vi "testTestCaseExecuted.vi"() -> (0 "error out":errorcluster)   [LabVIEW 2017, in "TestSuite.Tests.lvlib" / "Run.lvlib"]
uses:
  Run.lvlib
  TestSuite/TestSuite.lvclass
  TestResult/TestResult.lvclass
  Support/TestCaseMock/TestCaseMock.lvclass
  C:/Users/de200256/Code/logmanoriginal/lvunit/Test/Test.lvclass
  Assertion/Assertion.lvlib
  Test/Test.lvclass
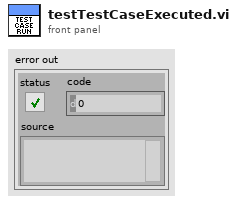
[diagram p1: front panel]
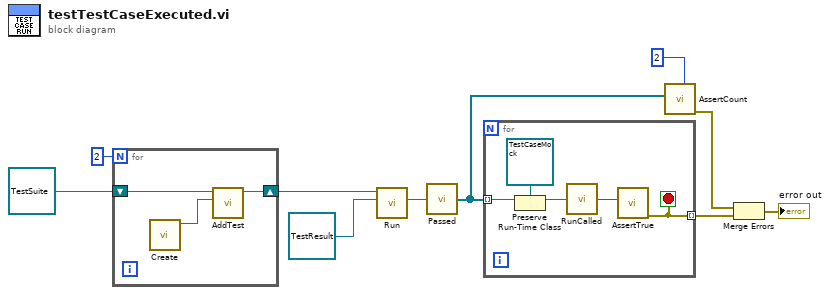
[diagram p0: block diagram]
diagram:
  n1 = for {
    N: 2 -> [_]
    shift-right: [w12] -> w8
    shift-left: refnum<class "TestSuite.lvclass"> refnum ("TestSuite.lvclass") -> [w13]
    n2 = call "Create.vi"() -> ("TestCaseMock"=w11:refnum<class "TestCaseMock.lvclass">)  [unwired: 10 in, 1 out]
    n3 = call-dynamic "AddTest.vi"("Test"=w11, "TestSuite in"=w13) -> ("TestSuite out"=w12:refnum<class "TestSuite.lvclass">)  [unwired: 8 in, 1 out]
  }
  n4 = call-dynamic "Run.vi"("TestResult"=refnum<class "TestResult.lvclass"> refnum ("TestResult.lvclass"), "TestSuite in"=w8) -> ("TestResult out"=w6:refnum<class "TestResult.lvclass">)  [unwired: 7 in, 2 out]
  n5 = call "Passed.vi"("TestResult In"=w6) -> ("Passed"=w2:refnum<class "Test.lvclass">[])
  n6 = for {
    tunnel: w2 -> [w18] mode=indexing
    tunnel: [w14] -> w5 mode=indexing
    stop <- w14 stop-if-true
    n7 = Preserve Run-Time Class(object in=w18, 2:refnum<class "TestCaseMock.lvclass"> refnum ("TestCaseMock")) -> (object out=w16:refnum<class "TestCaseMock.lvclass">)  [unwired: 1 in, 1 out]
    n8 = call "RunCalled.vi"("TestCaseMock In"=w16) -> ("Run Called"=w15:bool)
    n9 = call "AssertTrue.vi"("Condition"=w15) -> ("error out"=w14:errorcluster)  [unwired: 10 in]
  }
  n10 = call "AssertCount.vi"("Expected"=2, "Haystack"=w2) -> ("error out"=w3:errorcluster)  [unwired: 9 in]
  n11 = Merge Errors(w3, w5) -> (→"error out":errorcluster)
